vi "Count Only Once.vi"(1 "InValue":bool) -> (0 "Result":bool)   [LabVIEW 2015]
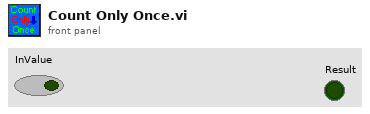
[diagram p1: front panel]
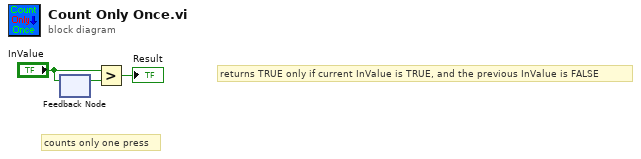
[diagram p0: block diagram]
diagram:
  # "returns TRUE only if current InValue is TRUE, and the previous InValue is FALSE"
  # "counts only one press"
  n1 = feedback #1() -> (w2:bool)  [unwired: 1 in]
  n2 = feedback-in #1("InValue") -> ()
  n3 = Greater?(x="InValue", y=w2) -> (0:→"Result":bool)
